vi "Ultrasonic Begin.vi"(8 "error in":errorcluster) -> (0 "error out":errorcluster)   [LabVIEW 2014]
uses:
  <vilib>/Rock Robotics/SystemInterfaces/AI/FPGA_AIChannel.ctl
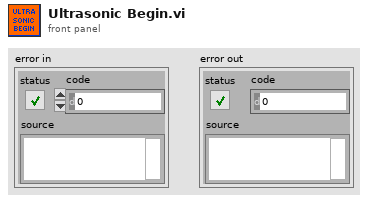
[diagram p1: front panel]
types:
  T1 = typedef "FPGA_AIChannel.ctl" = enum8{"AI 0", "AI 1", "AI 2", "AI 3", "AI MXP 0", "AI MXP 1", "AI MXP 2", "AI MXP 3", "Invalid"}
  T2 = typedef "WPI_AnalogChannelDevRef.ctl" = cluster{"DevStatus":errorcluster, "Controller":T3, "Analog Channel":T1}
  T3 = typedef "FPGA_TypedefAnalogModule.ctl" = enum16{"Controller 1"}
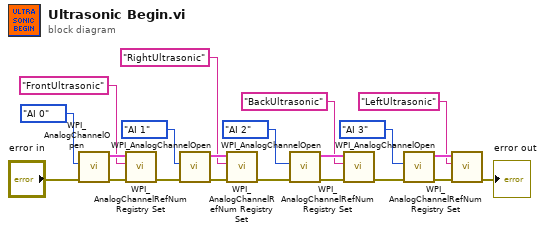
[diagram p0: block diagram]
diagram:
  n1 = call <vilib>:"WPI_AnalogChannelOpen.vi"("error in (no error)"="error in", "Analog Channel"=FPGA_AIChannel."AI 0") -> ("error out"=w7:errorcluster, "AIDeviceRef"=w8:T2)  [unwired: 8 in]
  n2 = call <vilib>:"WPI_AnalogChannelRefNum Registry Set.vi"("error in (no error)"=w7, "refnum name"="FrontUltrasonic", "AIDeviceRef"=w8) -> ("error out"=w12:errorcluster)  [unwired: 7 in, 1 out]
  n3 = call <vilib>:"WPI_AnalogChannelOpen.vi"("error in (no error)"=w12, "Analog Channel"=FPGA_AIChannel."AI 1") -> ("error out"=w10:errorcluster, "AIDeviceRef"=w9:T2)  [unwired: 8 in]
  n4 = call <vilib>:"WPI_AnalogChannelRefNum Registry Set.vi"("error in (no error)"=w10, "refnum name"="RightUltrasonic", "AIDeviceRef"=w9) -> ("error out"=w20:errorcluster)  [unwired: 7 in, 1 out]
  n5 = call <vilib>:"WPI_AnalogChannelOpen.vi"("error in (no error)"=w20, "Analog Channel"=FPGA_AIChannel."AI 2") -> ("error out"=w18:errorcluster, "AIDeviceRef"=w17:T2)  [unwired: 8 in]
  n6 = call <vilib>:"WPI_AnalogChannelRefNum Registry Set.vi"("error in (no error)"=w18, "refnum name"="BackUltrasonic", "AIDeviceRef"=w17) -> ("error out"=w13:errorcluster)  [unwired: 7 in, 1 out]
  n7 = call <vilib>:"WPI_AnalogChannelOpen.vi"("error in (no error)"=w13, "Analog Channel"=FPGA_AIChannel."AI 3") -> ("error out"=w15:errorcluster, "AIDeviceRef"=w16:T2)  [unwired: 8 in]
  n8 = call <vilib>:"WPI_AnalogChannelRefNum Registry Set.vi"("error in (no error)"=w15, "refnum name"="LeftUltrasonic", "AIDeviceRef"=w16) -> ("error out"=→"error out":errorcluster)  [unwired: 7 in, 1 out]
